vi "form_xyz_monitor.vi"(11 "JSON":string) -> ()   [LabVIEW 2021]
doc: "Form template VI.\n\nWhen you want to create a new form, please copy and modify this VI.\nThe form vi should be placed in the host/form directory."
uses:
  core/host_global_vars.vi
  <vilib>/Utility/error.llb/Error Cluster From Error Code.vi
  <vilib>/rvi/errors/niLvFpgaAdjustHostInterfaceError.vi
  <vilib>/rvi/interface/nirviReadWriteControl/nirviReadWriteControl.xnode
  FPGA Bitfiles/openlabspm_FPGATarget_fpgamain_eo-gUZR5D1g.lvbitx
  fpga/fpga_main.vi
  NiFpgaLv.dll
panel:
  out "XY Graph":cluster{sgl[], sgl[]}(graph)
  out "z (AO2)":u8(slide) scale=0.0..100.0
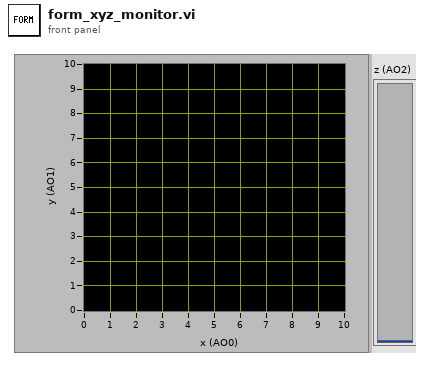
[diagram p1: front panel]
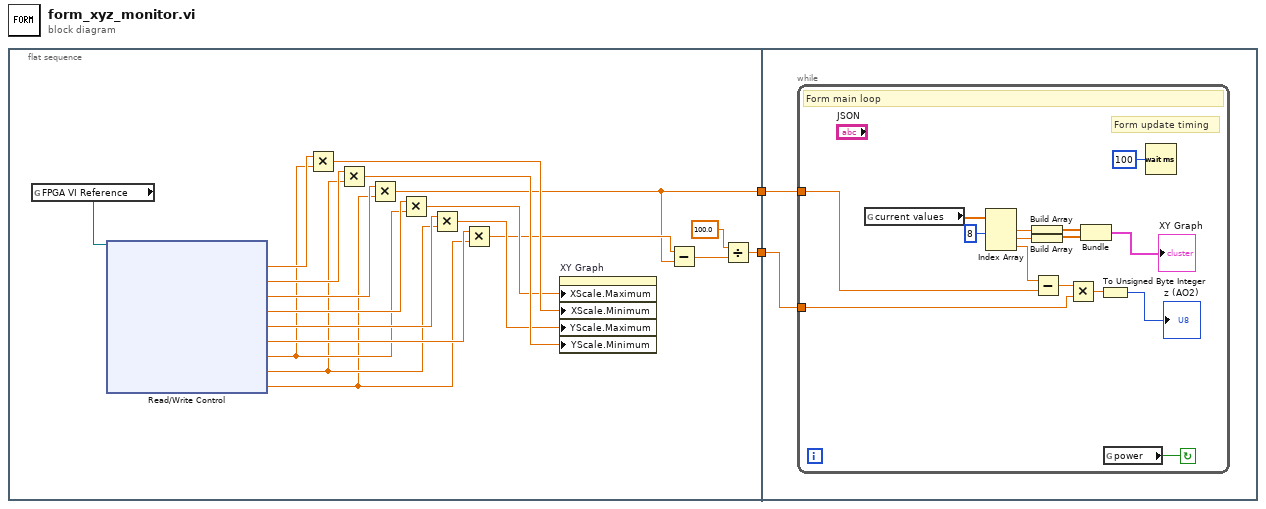
[diagram p0: block diagram]
diagram:
  n1 = flat-sequence {
    tunnel: [w6] -> w2
    tunnel: [w3] -> w1
    tunnel: w2 -> [w23]
    tunnel: w1 -> [w22]
    frame #0 {
      n2 = global read "host_global_vars.vi" "FPGA VI Reference"() -> (w21:refnum<k20>)
      n3 = xnode "Read/Write Control"("FPGA VI Reference In"=w21) -> ("limit (low, 10 V).ch 0"=w20:sgl, "limit (low, 10 V).ch 1"=w19:sgl, "limit (low, 10 V).ch 2"=w18:sgl, "limit (high, 10 V).ch 0"=w17:sgl, "limit (high, 10 V).ch 1"=w16:sgl, "limit (high, 10 V).ch 2"=w15:sgl, "ao gain.ch 0"=w14:sgl, "ao gain.ch 1"=w13:sgl, "ao gain.ch 2"=w12:sgl)  [unwired: 1 in, 2 out]
      n4 = Multiply(x=w20, y=w14) -> (x*y=w11:sgl)
      n5 = Multiply(x=w19, y=w13) -> (x*y=w10:sgl)
      n6 = Multiply(x=w18, y=w12) -> (x*y=w6:sgl)
      n7 = Multiply(x=w17, y=w14) -> (x*y=w9:sgl)
      n8 = Multiply(x=w16, y=w13) -> (x*y=w8:sgl)
      n9 = Multiply(x=w15, y=w12) -> (x*y=w7:sgl)
      n10 = property on="XY Graph" class="XYGraph (strict)"("XScale.Maximum"=w9, "XScale.Minimum"=w11, "YScale.Maximum"=w8, "YScale.Minimum"=w10) -> ()  [unwired: 2 in, 2 out]
      n11 = Subtract(x=w7, y=w6) -> (x-y=w5:sgl)
      n12 = Divide(x=100.0, y=w5) -> (x/y=w3:dbl)
    }
    frame #1 {
      n13 = while {
        tunnel: w23 -> [w29]
        tunnel: w22 -> [w27]
        stop <- w38 continue-if-true
        # "Form update timing"
        # "Form main loop"
        n14 = global read "host_global_vars.vi" "current values"() -> (w36:sgl[])
        n15 = Index Array(array=w36, index #1=8 ("index")) -> (element #1=w35:sgl, element #2=w32:sgl, element #3=w30:sgl)  [unwired: 2 in]
        n16 = Build Array(w35) -> (w34:sgl[])
        n17 = Build Array(w32) -> (w33:sgl[])
        n18 = Subtract(x=w30, y=w29) -> (x-y=w28:sgl)
        n19 = Multiply(x=w28, y=w27) -> (x*y=w26:dbl)
        n20 = Bundle(w34, w33) -> (→"XY Graph":cluster{sgl[], sgl[]})  [unwired: 1 in]
        n21 = To Unsigned Byte Integer(number=w26) -> (unsigned 8bit integer=→"z (AO2)":u8)
        n22 = global read "host_global_vars.vi" "power"() -> (w38:bool)
        n23 = Wait (ms)(milliseconds to wait=u32 100) -> ()  [unwired: 1 out]
      }
    }
  }
